vi "NI-Switch Global.vi"() -> ()   [LabVIEW 2010, in "NI-Switch Relay Custom Device.lvlib"]
uses:
  NI-Switch Relay Custom Device.lvlib
panel:
  in  "Main Prop Names":string[](array[string])=["Physical Address", "Topology Name"]
  in  "Relay Prop. Names":string[](array[string])=["Relay Name"]
  in  "Dig Out":string="Digital Output"
  in  "Relay Ch GUID":string="6DEB9409-FEEE-79F6-ED3C-247B42A52503"
  in  "Relay Ch":string="Relay Channel"
  in  "Sub Relay GUID":string="3D447138-A707-99DE-4D8F-561BC6A270C2"
  in  "Sub Relay":string="Relays"
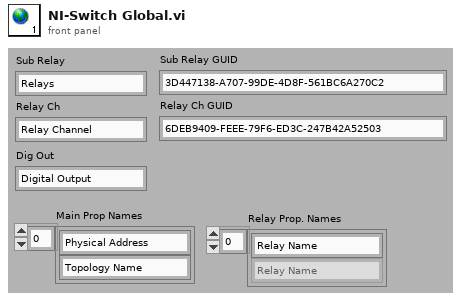
[diagram p1: front panel]
diagram:
